vi "Run JSL (File).vi"(8 "error in (no error)":errorcluster, 10 "JSL file":path, 11 "JMP application":refnum<k7>) -> (0 "error out":errorcluster, 3 "JMP application out":refnum<k7>)   [LabVIEW 2019, in "JMP Automation.lvlib"]
doc: "Loads a JSL text file from disk given a valid path name, and then submits the text for execution\nwithin JMP"
uses:
  JMP Automation.lvlib
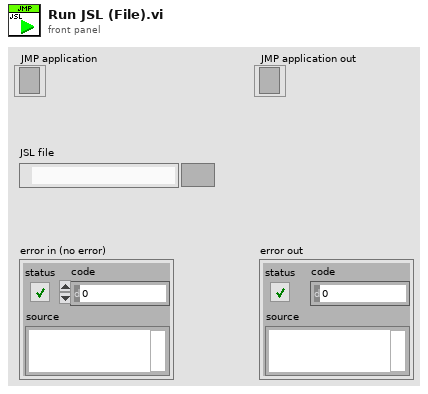
[diagram p1: front panel]
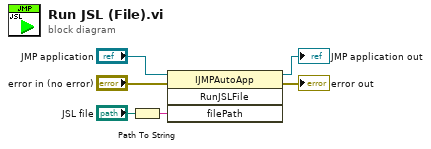
[diagram p0: block diagram]
diagram:
  n1 = Path To String(path="JSL file") -> (string=w1:string)
  n2 = invoke class="IJMPAutoApp" method="RunJSLFile"(reference="JMP application", error in="error in (no error)", "filePath"=w1) -> (reference out=→"JMP application out":refnum<k7>, error out=→"error out":errorcluster)  [unwired: 1 in, 2 out]
